vi "Write preset modes.vi"(8 "error in (no error)":errorcluster, 10 "preset modes":T1, 11 "S4GEI in":refnum<class "S4GEI.lvclass">) -> (0 "error out":errorcluster, 3 "S4GEI out":refnum<class "S4GEI.lvclass">)   [LabVIEW 2018, in "S4GEI.lvclass"]
uses:
  S4GEI.lvclass
  S4GEI.lvclass/S4GEI.ctl
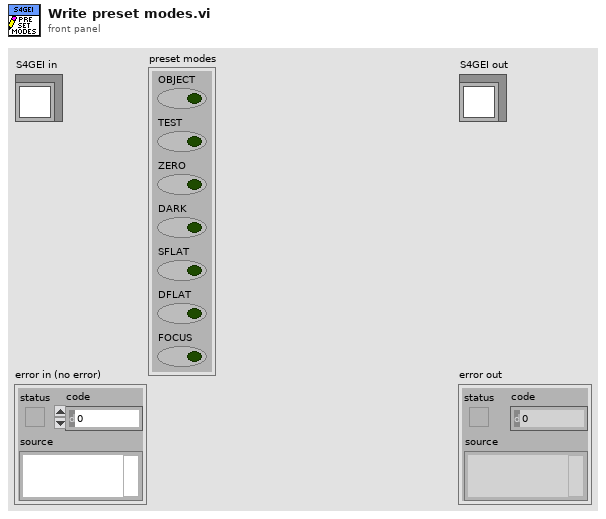
[diagram p1: front panel]
types:
  T1 = cluster{"OBJECT":bool, "TEST":bool, "ZERO":bool, "DARK":bool, "SFLAT":bool, "DFLAT":bool, "FOCUS":bool}
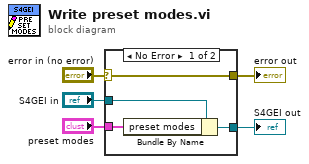
[diagram p0: block diagram]
diagram:
  n1 = case shown="No Error" "error in (no error)" {
    selector: "error in (no error)" -> [w9 w10]
    tunnel: [w9 w10] -> w4
    tunnel: [w7 w11] -> w2
    tunnel: "S4GEI in" -> [w8 w11]
    tunnel: "preset modes" -> [w6 _]
    frame No Error {
      n2 = Bundle By Name(cluster=w8, "preset modes"=w6) -> (w7:refnum<class "S4GEI.lvclass">)
    }
    frame Error {
    }
  }
  "error out" <- w4
  "S4GEI out" <- w2
